vi "20150813 multi servo control.vi"() -> ()   [LabVIEW 2013]
uses:
  <vilib>/MakerHub/LINX/Public/Sensors/Motion/Servo/Servo Open N Channels.vi
  <vilib>/MakerHub/LINX/Public/Sensors/Motion/Servo/Servo Close N Channels.vi
  <vilib>/MakerHub/LINX/Public/Sensors/Motion/Servo/Servo Set Pulse Width N Channels.vi
  <vilib>/MakerHub/LINX/LMH-LINX.lvlib
  <vilib>/MakerHub/LINX/Public/Sensors/Motion/Servo/Servo.lvlib
panel:
  in  "Pulse Widths (uS)":u16[](array[numeric])=[1500, 1500, 1500, 1500, 1500, 1500, 1500, 1500, 1500, 1500, 1500, 1600] min=600 max=2400 step=100
  in  "Servo Channels":u8[](array[numeric])=[2, 3, 4, 5, 6, 7, 8, 9, 10, 11, 12, 13]
  in  "error in (no error)":errorcluster
  out "Error Out":errorcluster
  out "Initialize OK?":bool=TRUE
  in  "Stop Button":bool
  in  "Serial Port":refnum<visa-resource-name>="COM10"
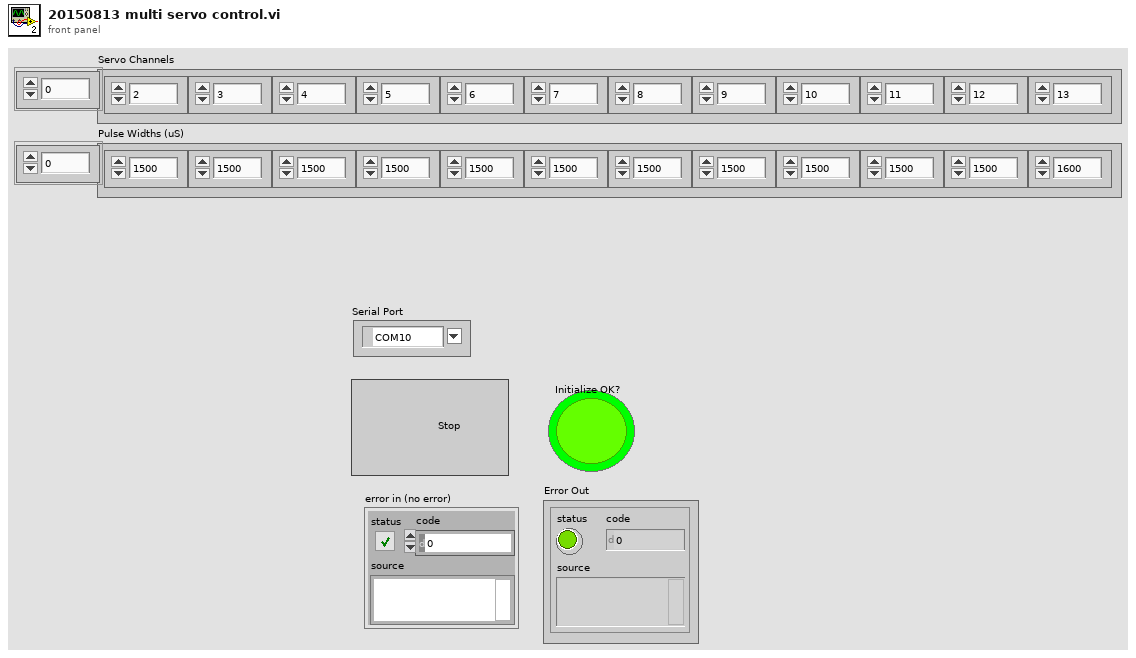
[diagram p1: front panel]
types:
  T1 = typedef "LMH-LINX.lvlib/LINX Ref.ctl" = cluster{"Platform":T2, "Interface":T3, "LINX Device Config":T4}
  T2 = typedef "LMH-LINX.lvlib/Platform.ctl" = enum16{"LINX", "myRIO"}
  T3 = typedef "LMH-LINX.lvlib/Interface.ctl" = enum16{"Serial", "TCP"}
  T4 = typedef "LMH-LINX.lvlib/Device.lvlib/LINX Device Config.ctl" = cluster{"Interface":T3, "COM Port":refnum<visa-resource-name>, "TCP Configuration":T5, "Device Family":u8, "Device ID":u8, "Device Name":string, "TCP Ref":refnum<k5>, "Channels":T6}
  T5 = typedef "LMH-LINX.lvlib/Device.lvlib/TCP Config.ctl" = cluster{"IP Address":string, "Port":u16}
  T6 = typedef "LMH-LINX.lvlib/Channels.ctl" = cluster{"DI":u8[], "DO":u8[], "AI":u8[], "AO":u8[], "PWM":u8[], "QE":u8[], "UART":u8[], "I2C 2":u8[], "SPI":u8[], "CAN":u8[], "Servo":u8[], "AI Ref (V)":dbl, "AO Ref (V)":dbl, "AO Resolution (Bits)":u8}
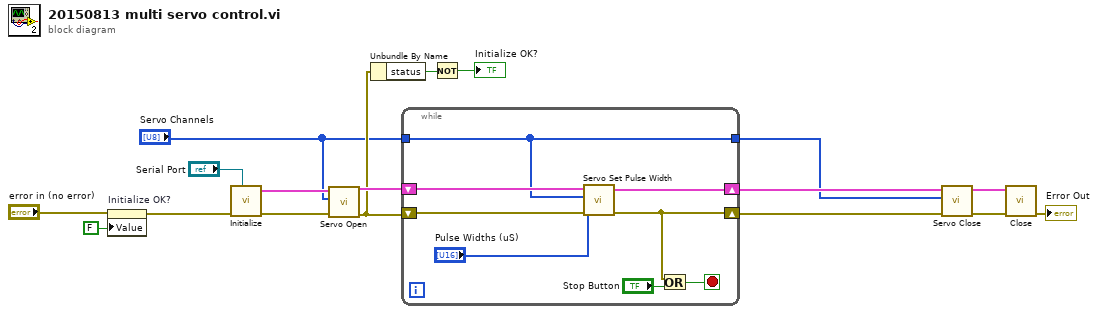
[diagram p0: block diagram]
diagram:
  n1 = property on="Initialize OK?" class="Bool (strict)"(error in="error in (no error)", "Value"=FALSE ("Initialize OK?")) -> (error out=w6:errorcluster)  [unwired: 1 in, 1 out]
  n2 = call <vilib>:"Initialize.vi"("Serial Port"="Serial Port", "Error In"=w6) -> ("Error Out"=w16:errorcluster, "LINX Ref"=w15:T1)  [unwired: 7 in, 1 out]
  n3 = call-poly <vilib>:"Servo Open.vi"("Error In"=w16, "Servo Channels"="Servo Channels", "LINX Resource"=w15) -> ("Error Out"=w9:errorcluster, "LINX Resource"=w14:T1)  [unwired: 7 in]
  n4 = Unbundle By Name(w9) -> ("status"=w8:bool)
  n5 = while {
    shift-right: [w22] -> w10
    shift-left: w9 -> [w23]
    tunnel: "Servo Channels" -> [w19]
    shift-right: [w20] -> w13
    shift-left: w14 -> [w21]
    tunnel: [w19] -> w1
    stop <- w25 stop-if-true
    n6 = call-poly <vilib>:"Servo Set Pulse Width.vi"("Error In"=w23, "Pulse Widths (uS)"="Pulse Widths (uS)", "Servo Channels"=w19, "LINX Resource"=w21) -> ("Error Out"=w22:errorcluster, "LINX Resource"=w20:T1)  [unwired: 6 in]
    n7 = Or(x=w22, y="Stop Button") -> (x .or. y?=w25:bool)
  }
  n8 = Not(x=w8) -> (.not. x?=→"Initialize OK?":bool)
  n9 = call-poly <vilib>:"Servo Close.vi"("Error In"=w10, "Servo Channels"=w1, "LINX Resource"=w13) -> ("Error Out"=w11:errorcluster, "LINX Resource"=w12:T1)  [unwired: 7 in]
  n10 = call <vilib>:"Close.vi"("Error In"=w11, "LINX Resource"=w12) -> ("Error Out"=→"Error Out":errorcluster)  [unwired: 8 in, 1 out]
